vi "SETI_LV_FGV.vi"(0 "NumDataPoints in":i32, 1 "Command":T2, 5 "DataIn in":csg[](array[numeric]), 7 "num_cfft in":i32, 9 "Chirp FFT Pairs in":T1[](array[typedef]), 11 "subband_sample_rate in":dbl) -> (4 "NumDataPoints out":i32, 6 "DataIn out":csg[](array[numeric]), 8 "num_cfft out":i32, 10 "Chirp FFT Pairs out":T1[](array[typedef]), 15 "subband_sample_rate out":dbl)   [LabVIEW 2015, in "SETI_LV.lvlib"]
uses:
  SETI_LV.lvlib
  SETI_LV_FGV.ctl
  TypeDefs/ChirpFFT Pairs.ctl
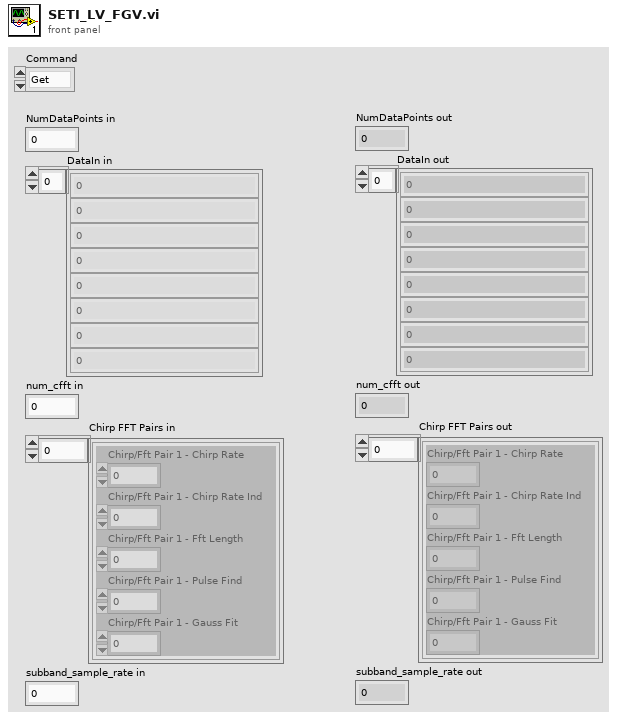
[diagram p1: front panel]
types:
  T1 = typedef "SETI_LV.lvlib/ChirpFFT Pairs.ctl" = cluster{"Chirp/Fft Pair 1 - Chirp Rate":dbl, "Chirp/Fft Pair 1 - Chirp Rate Ind":i32, "Chirp/Fft Pair 1 - Fft Length":i32, "Chirp/Fft Pair 1 - Pulse Find":i32, "Chirp/Fft Pair 1 - Gauss Fit":i32}
  T2 = typedef "SETI_LV.lvlib/SETI_LV_FGV.ctl" = enum16{"Get", "Set", "Chirp(icfft)"}
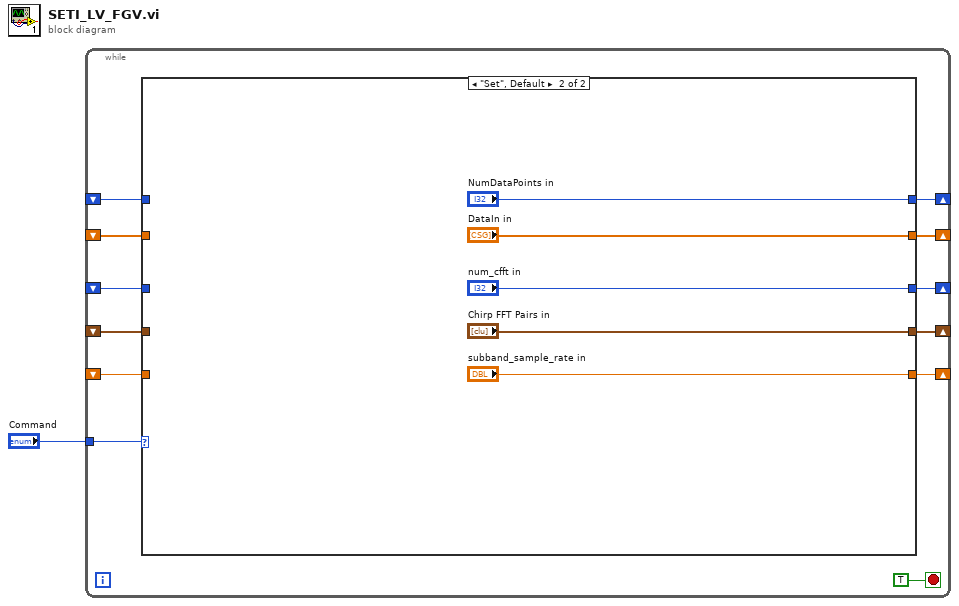
[diagram p0: block diagram]
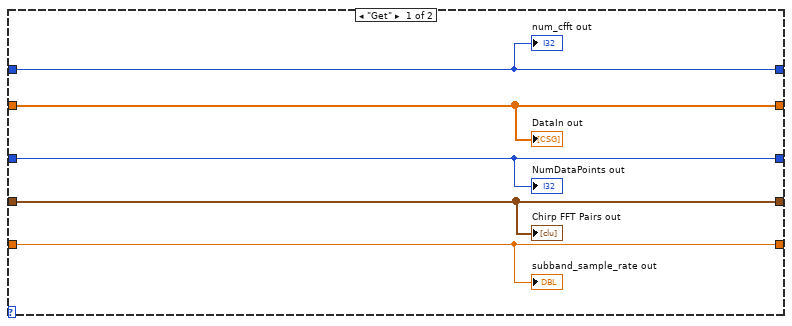
[diagram p2: hidden frame]
diagram:
  n1 = while {
    tunnel: "Command" -> [w12]
    shift-right: [w11] -> _
    shift-left: _ -> [w6]
    shift-right: [w10] -> _
    shift-left: _ -> [w5]
    shift-right: [w9] -> _
    shift-left: _ -> [w4]
    shift-right: [w8] -> _
    shift-left: _ -> [w3]
    shift-right: [w7] -> _
    shift-left: _ -> [w2]
    stop <- TRUE stop-if-true
    n2 = case shown="\"Set\", Default" w12 {
      tunnel: [w18 "NumDataPoints in"] -> w11
      tunnel: [w17 "DataIn in"] -> w10
      tunnel: [w16 "num_cfft in"] -> w9
      tunnel: [w15 "Chirp FFT Pairs in"] -> w8
      tunnel: [w14 "subband_sample_rate in"] -> w7
      tunnel: w6 -> [w18 _]
      tunnel: w5 -> [w17 _]
      tunnel: w4 -> [w16 _]
      tunnel: w3 -> [w15 _]
      tunnel: w2 -> [w14 _]
      frame "Get" {
        "subband_sample_rate out" <- w14
        "num_cfft out" <- w18
        "DataIn out" <- w17
        "Chirp FFT Pairs out" <- w15
        "NumDataPoints out" <- w16
      }
      frame "Set", Default {
      }
    }
  }
